vi "Set Port Database.vi"(8 "error in":errorcluster, 9 "Database Path":path, 10 "Database Name":string, 11 "Port Ref":T1 format="%.0x") -> (0 "error out":errorcluster, 3 "Port Ref out":T1 format="%.0x")   [LabVIEW 2020, in "Ballard MIL-STD-1553 Scripting.lvlib"]
uses:
  Ballard MIL-STD-1553 Scripting.lvlib
  <vilib>/NI VeriStand/Custom Device API/Custom Device Item Ref.ctl
  Constants.vi
  <vilib>/NI VeriStand/Custom Device API/Set Item Property (String).vi
  <vilib>/NI VeriStand/Custom Device API/Set Item Property (Path).vi
  <vilib>/NI VeriStand/Custom Device API/Custom Device API.lvlib
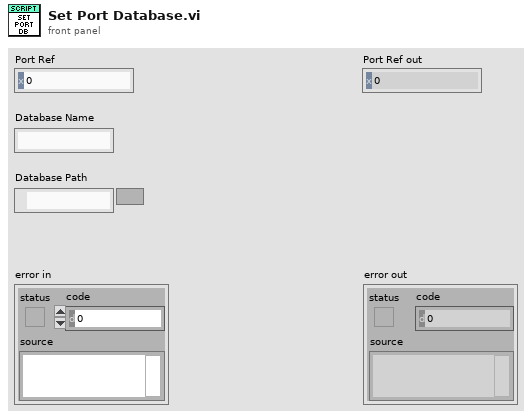
[diagram p1: front panel]
types:
  T1 = typedef "Custom Device API.lvlib/Custom Device Item Ref.ctl" = u64
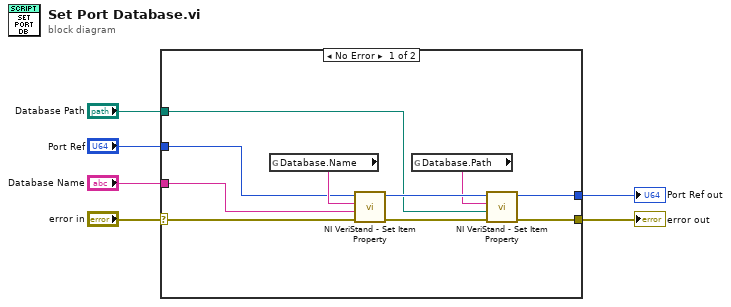
[diagram p0: block diagram]
diagram:
  n1 = case shown="No Error" "error in" {
    selector: "error in" -> [w7 w18]
    tunnel: "Port Ref" -> [w10 w17]
    tunnel: [w16 w18] -> w5
    tunnel: "Database Name" -> [w9 _]
    tunnel: "Database Path" -> [w8 _]
    tunnel: [w15 w17] -> w2
    frame No Error {
      n2 = global read "Constants.vi" "Database.Name"() -> (w11:string)
      n3 = call-poly <vilib>:"NI VeriStand - Set Item Property.vi"("error in (no error)"=w7, "Value"=w9, "Property Name"=w11, "Item Ref in"=w10) -> ("error out"=w13:errorcluster, "Item Ref out"=w14:T1)  [unwired: 5 in, 1 out]
      n4 = global read "Constants.vi" "Database.Path"() -> (w12:string)
      n5 = call-poly <vilib>:"NI VeriStand - Set Item Property.vi"("error in (no error)"=w13, "Value"=w8, "Property Name"=w12, "Item Ref in"=w14) -> ("error out"=w16:errorcluster, "Item Ref out"=w15:T1)  [unwired: 5 in, 1 out]
    }
    frame Error {
    }
  }
  "error out" <- w5
  "Port Ref out" <- w2
